vi "CRYWindow WAIT PROJECT OPEN.vi"   [LabVIEW 2013]
uses:
  CRYProject/CRYProject Editor Global.vi
panel:
  # "Wait Until Project is Load...."
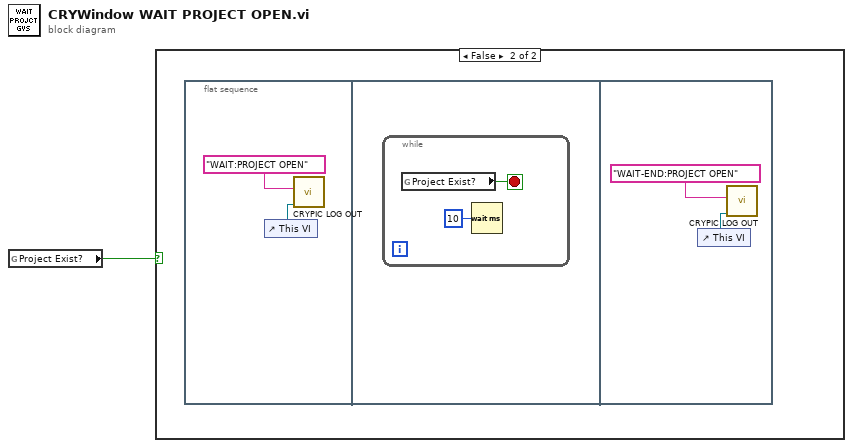
[diagram p0: block diagram]
diagram:
  n1 = global read "CRYProject Editor Global.vi" "Project Exist?"() -> (w1:bool)
  n2 = case shown="False" w1 {
    frame True {
    }
    frame False {
      n3 = flat-sequence {
        frame #0 {
          n4 = control-ref of="This VI"() -> (w3:refnum<vi>)
          n5 = call "CRYPIC LOG OUT.vi"("pVIRef"=w3, "sData"="WAIT:PROJECT OPEN" ("format string")) -> ()  [unwired: 10 in]
        }
        frame #1 {
          n6 = while {
            stop <- w5 stop-if-true
            n7 = global read "CRYProject Editor Global.vi" "Project Exist?"() -> (w5:bool)
            n8 = Wait (ms)(milliseconds to wait=u32 10) -> ()  [unwired: 1 out]
          }
        }
        frame #2 {
          n9 = control-ref of="This VI"() -> (w6:refnum<vi>)
          n10 = call "CRYPIC LOG OUT.vi"("pVIRef"=w6, "sData"="WAIT-END:PROJECT OPEN" ("format string")) -> ()  [unwired: 10 in]
        }
      }
    }
  }
